vi "DashboardGetvi.vi"(8 "Joystick 2":T1, 9 "Joystick 1":T1) -> ()   [LabVIEW 2018]
uses:
  <vilib>/Rock Robotics/WPI/Joystick/WPI_JoystickDevRef.ctl
  <vilib>/Rock Robotics/WPI/Joystick/WPI_JoystickDeviceEnum.ctl
  <vilib>/Rock Robotics/Network Tables/NT Read Boolean.vi
  <vilib>/Rock Robotics/Network Tables/NT Read Number.vi
  Inputs_DriverStation.vi
  RobotStates.vi
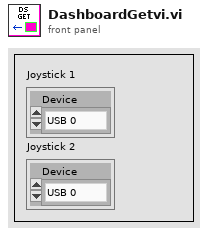
[diagram p1: front panel]
types:
  T1 = typedef "WPI_JoystickDevRef.ctl" = cluster{"Device":T2}
  T2 = typedef "WPI_JoystickDeviceEnum.ctl" = enum16{"USB 0", "USB 1", "USB 2", "USB 3", "USB 4", "USB 5"}
  T3 = cluster{bool, bool, bool, bool, bool, bool, bool, bool, bool, bool, bool, bool, bool, bool}
  T4 = cluster{"Boolean":bool, "Boolean":bool, "Boolean":bool, "Boolean":bool, "Boolean":bool, "Boolean":bool, "Boolean":bool, "Boolean":bool, "Boolean":bool, "Boolean":bool, "Boolean":bool, "Boolean":bool, "Boolean":bool, "Boolean":bool}
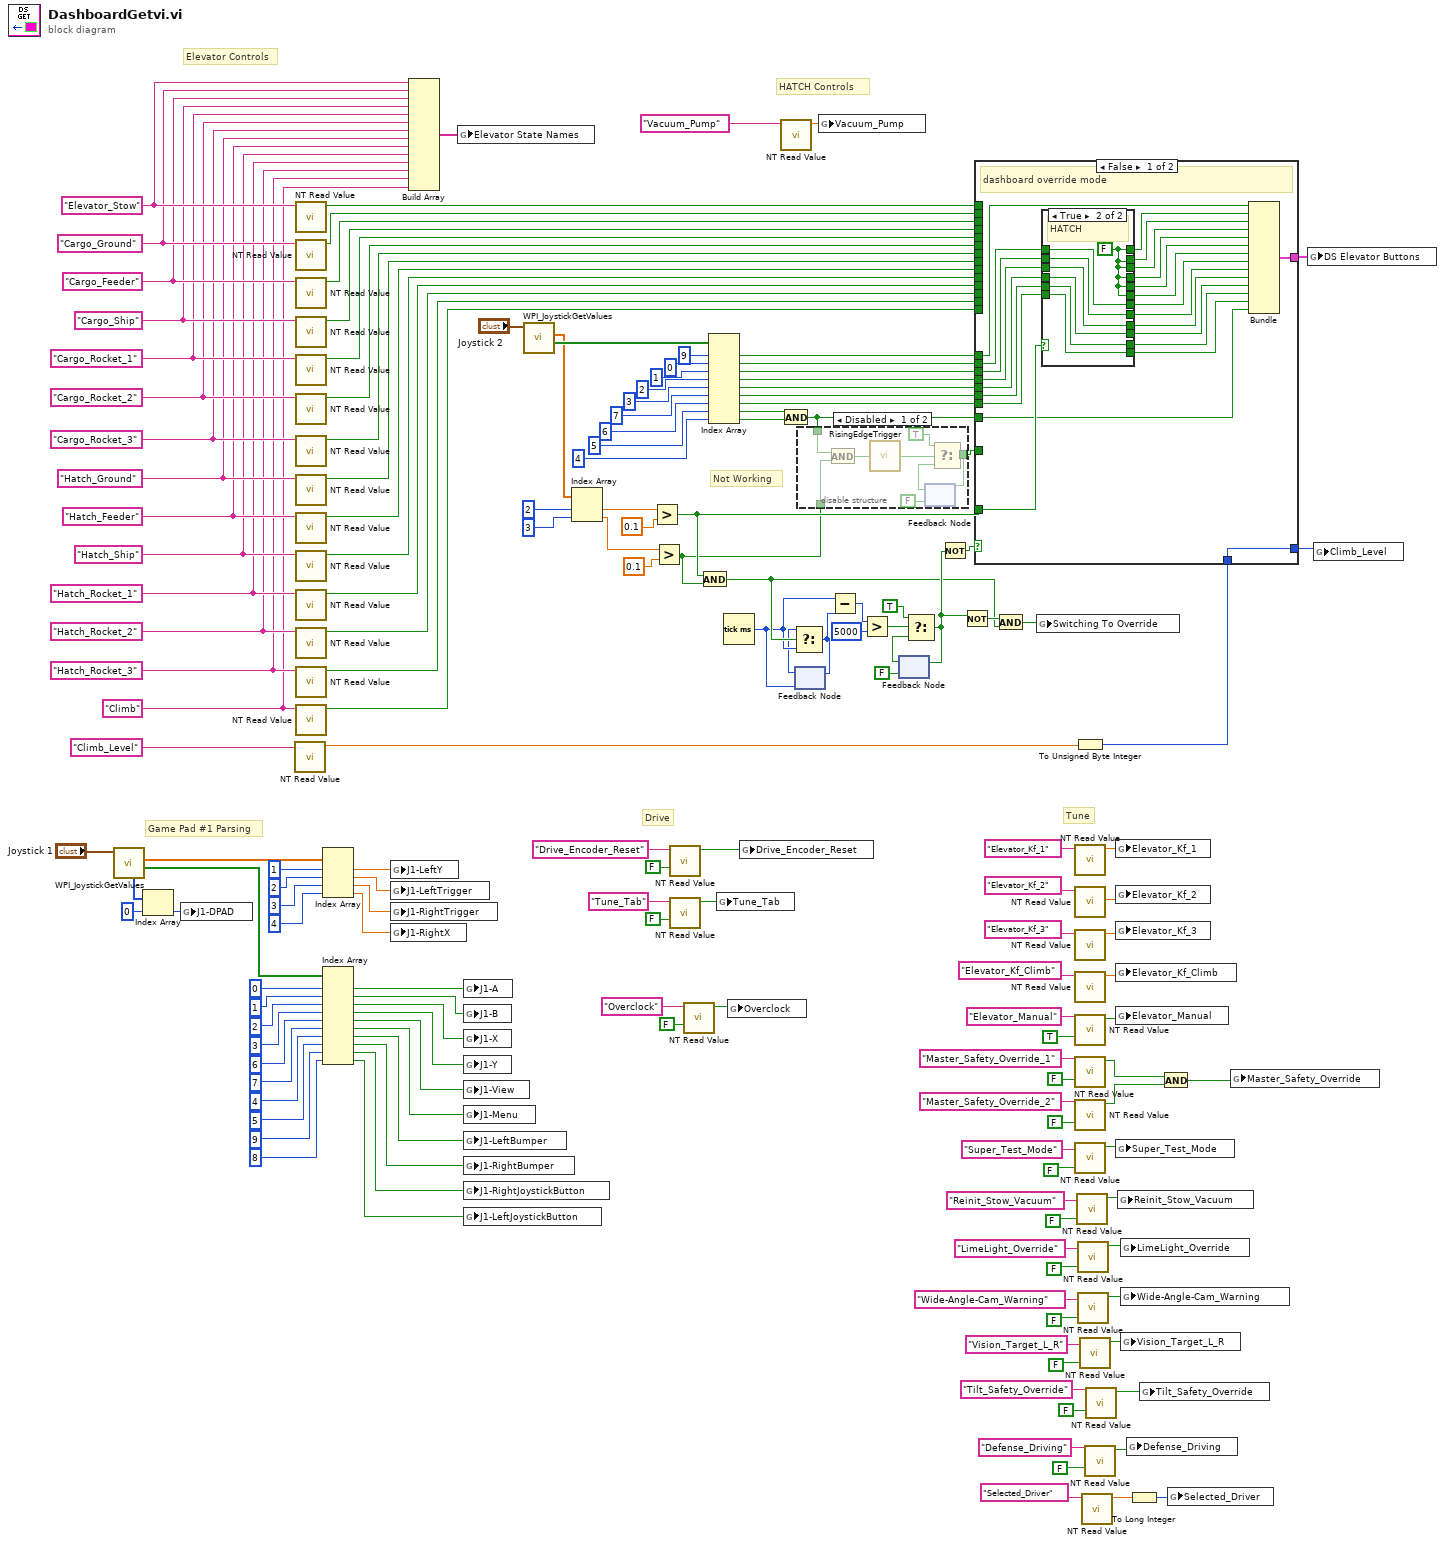
[diagram p0: block diagram]
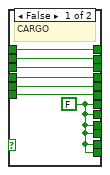
[diagram p3: hidden frame]
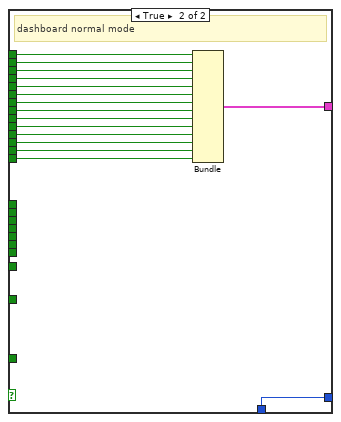
[diagram p4: hidden frame]
diagram:
  w95 = "Climb" ("refnum name")
  w103 = "Hatch_Rocket_3" ("refnum name")
  w104 = "Hatch_Rocket_2" ("refnum name")
  w105 = "Hatch_Rocket_1" ("refnum name")
  w106 = "Hatch_Ship" ("refnum name")
  w107 = "Hatch_Feeder" ("refnum name")
  w108 = "Hatch_Ground" ("refnum name")
  w152 = "Cargo_Rocket_3" ("refnum name")
  w153 = "Cargo_Rocket_2" ("refnum name")
  w154 = "Cargo_Rocket_1" ("refnum name")
  w155 = "Cargo_Ship" ("refnum name")
  w161 = "Cargo_Feeder" ("refnum name")
  w162 = "Cargo_Ground" ("refnum name")
  w163 = "Elevator_Stow" ("refnum name")
  # "Not Working"
  # "Tune"
  # "Drive"
  # "HATCH Controls"
  # "Game Pad #1 Parsing"
  # "Elevator Controls"
  n1 = call <vilib>:"WPI_JoystickGetValues.vi"("JoystickDevRef"="Joystick 1") -> ("Buttons"=w143:bool[], "Axes"=w142:dbl[], "POVs"=w139:i16[])  [unwired: 6 in, 2 out]
  n2 = Index Array(array=w139, index=0) -> (element=w136:i16)
  n3 = global write "Inputs_DriverStation.vi" "J1-DPAD"(w136) -> ()
  n4 = call-poly <vilib>:"NT Read Value.vi"("Name"="Climb_Level" ("refnum name")) -> ("Numeric"=w12:dbl)  [unwired: 9 in, 1 out]
  n5 = call-poly <vilib>:"NT Read Value.vi"("Name"=w163) -> ("Boolean"=w166:bool)  [unwired: 9 in, 1 out]
  n6 = call-poly <vilib>:"NT Read Value.vi"("Name"=w162) -> ("Boolean"=w165:bool)  [unwired: 9 in, 1 out]
  n7 = call-poly <vilib>:"NT Read Value.vi"("Name"=w161) -> ("Boolean"=w164:bool)  [unwired: 9 in, 1 out]
  n8 = call-poly <vilib>:"NT Read Value.vi"("Name"=w155) -> ("Boolean"=w159:bool)  [unwired: 9 in, 1 out]
  n9 = call-poly <vilib>:"NT Read Value.vi"("Name"=w154) -> ("Boolean"=w158:bool)  [unwired: 9 in, 1 out]
  n10 = call-poly <vilib>:"NT Read Value.vi"("Name"=w153) -> ("Boolean"=w157:bool)  [unwired: 9 in, 1 out]
  n11 = call-poly <vilib>:"NT Read Value.vi"("Name"=w152) -> ("Boolean"=w156:bool)  [unwired: 9 in, 1 out]
  n12 = call-poly <vilib>:"NT Read Value.vi"("Name"=w108) -> ("Boolean"=w115:bool)  [unwired: 9 in, 1 out]
  n13 = call-poly <vilib>:"NT Read Value.vi"("Name"=w107) -> ("Boolean"=w114:bool)  [unwired: 9 in, 1 out]
  n14 = call-poly <vilib>:"NT Read Value.vi"("Name"=w106) -> ("Boolean"=w113:bool)  [unwired: 9 in, 1 out]
  n15 = call-poly <vilib>:"NT Read Value.vi"("Name"=w105) -> ("Boolean"=w112:bool)  [unwired: 9 in, 1 out]
  n16 = call-poly <vilib>:"NT Read Value.vi"("Name"=w104) -> ("Boolean"=w111:bool)  [unwired: 9 in, 1 out]
  n17 = call-poly <vilib>:"NT Read Value.vi"("Name"=w103) -> ("Boolean"=w110:bool)  [unwired: 9 in, 1 out]
  n18 = call-poly <vilib>:"NT Read Value.vi"("Name"=w95) -> ("Boolean"=w94:bool)  [unwired: 9 in, 1 out]
  n19 = Index Array(array=w142, index #1=1 ("index"), index #2=2 ("index"), index #3=3 ("index"), index #4=4 ("index")) -> (element #1=w129:dbl, element #2=w130:dbl, element #3=w131:dbl, element #4=w128:dbl)
  n20 = Index Array(array=w143, index #1=0 ("index"), index #2=1 ("index"), index #3=2 ("index"), index #4=3 ("index"), index #5=6 ("index"), index #6=7 ("index"), index #7=4 ("index"), index #8=5 ("index"), index #9=9 ("index"), index #10=8 ("index")) -> (element #1=w135:bool, element #2=w134:bool, element #3=w133:bool, element #4=w132:bool, element #5=w92:bool, element #6=w88:bool, element #7=w85:bool, element #8=w84:bool, element #9=w82:bool, element #10=w77:bool)
  n21 = global write "Inputs_DriverStation.vi" "J1-LeftY"(w129) -> ()
  n22 = global write "Inputs_DriverStation.vi" "J1-LeftTrigger"(w130) -> ()
  n23 = global write "Inputs_DriverStation.vi" "J1-RightTrigger"(w131) -> ()
  n24 = global write "Inputs_DriverStation.vi" "J1-RightX"(w128) -> ()
  n25 = Build Array(w163, w162, w161, w155, w154, w153, w152, w108, w107, w106, w105, w104, w103, w95) -> (w160:string[])
  n26 = global write "RobotStates.vi" "Elevator State Names"(w160) -> ()
  n27 = global write "Inputs_DriverStation.vi" "J1-A"(w135) -> ()
  n28 = global write "Inputs_DriverStation.vi" "J1-B"(w134) -> ()
  n29 = global write "Inputs_DriverStation.vi" "J1-X"(w133) -> ()
  n30 = global write "Inputs_DriverStation.vi" "J1-Y"(w132) -> ()
  n31 = global write "Inputs_DriverStation.vi" "J1-View"(w92) -> ()
  n32 = global write "Inputs_DriverStation.vi" "J1-Menu"(w88) -> ()
  n33 = global write "Inputs_DriverStation.vi" "J1-LeftBumper"(w85) -> ()
  n34 = global write "Inputs_DriverStation.vi" "J1-RightBumper"(w84) -> ()
  n35 = global write "Inputs_DriverStation.vi" "J1-RightJoystickButton"(w82) -> ()
  n36 = global write "Inputs_DriverStation.vi" "J1-LeftJoystickButton"(w77) -> ()
  n37 = call <vilib>:"WPI_JoystickGetValues.vi"("JoystickDevRef"="Joystick 2") -> ("Buttons"=w72:bool[], "Axes"=w56:dbl[])  [unwired: 6 in, 3 out]
  n38 = Index Array(array=w56, index #1=2 ("index"), index #2=3 ("index")) -> (element #1=w55:dbl, element #2=w51:dbl)
  n39 = Greater?(x=w55, y=0.1) -> (0:w50:bool)
  n40 = Greater?(x=w51, y=0.1) -> (0:w38:bool)
  n41 = call-poly <vilib>:"NT Read Value.vi"("Default Value"=FALSE, "Name"="Drive_Encoder_Reset" ("refnum name")) -> ("Boolean"=w116:bool)  [unwired: 8 in, 1 out]
  n42 = call-poly <vilib>:"NT Read Value.vi"("Default Value"=FALSE, "Name"="Tune_Tab" ("refnum name")) -> ("Boolean"=w79:bool)  [unwired: 8 in, 1 out]
  n43 = call-poly <vilib>:"NT Read Value.vi"("Default Value"=FALSE, "Name"="Overclock" ("refnum name")) -> ("Boolean"=w26:bool)  [unwired: 8 in, 1 out]
  n44 = And(x=w50, y=w38) -> (x .and. y?=w32:bool)
  n45 = Index Array(array=w72, index #1=9 ("index"), index #2=0 ("index"), index #3=1 ("index"), index #4=2 ("index"), index #5=3 ("index"), index #6=7 ("index"), index #7=6 ("index"), index #8=5 ("index"), index #9=4 ("index")) -> (element #1=w70:bool, element #2=w68:bool, element #3=w66:bool, element #4=w64:bool, element #5=w62:bool, element #6=w60:bool, element #7=w58:bool, element #8=w41:bool, element #9=w40:bool)
  n46 = global write "Inputs_DriverStation.vi" "Tune_Tab"(w79) -> ()
  n47 = Tick Count (ms)() -> (millisecond timer value=w30:u32)
  n48 = global write "Inputs_DriverStation.vi" "Overclock"(w26) -> ()
  n49 = global write "Inputs_DriverStation.vi" "Drive_Encoder_Reset"(w116) -> ()
  n50 = call-poly <vilib>:"NT Read Value.vi"("Name"="Vacuum_Pump" ("refnum name")) -> ("Numeric"=w119:dbl)  [unwired: 9 in, 1 out]
  n51 = And(x=w41, y=w40) -> (x .and. y?=w39:bool)
  n52 = feedback #1(w30) -> (w29:u32)
  n53 = Select(t=w29, s=w32, f=w30) -> (s? t:f=w36:u32)
  n54 = feedback-in #1(w36) -> ()
  n55 = disable-structure shown="Disabled" {
    disable-tunnel: w39 -> [w174 _]
    disable-tunnel: w38 -> [w173 _]
    disable-tunnel: [w167 _] -> w37
    frame Disabled {
      n56 = And(x=w174, y=w173) -> (x .and. y?=w172:bool)
      n57 = call "RisingEdgeTrigger.vi"("Raw Signal"=w172) -> ("Trigger"=w168:bool)
      n58 = feedback #2(FALSE) -> (w170:bool)
      n59 = Select(t=TRUE, s=w168, f=w170) -> (s? t:f=w167:bool)
      n60 = feedback-in #2(w167) -> ()
    }
    frame Enabled {
    }
  }
  n61 = global write "Inputs_DriverStation.vi" "Vacuum_Pump"(w119) -> ()
  n62 = Subtract(x=w30, y=w36) -> (x-y=w35:u32)
  n63 = Greater?(x=w35, y=u32 5000) -> (0:w48:bool)
  n64 = feedback #3(FALSE) -> (w46:bool)
  n65 = Select(t=TRUE, s=w48, f=w46) -> (s? t:f=w33:bool)
  n66 = feedback-in #3(w33) -> ()
  n67 = Not(x=w33) -> (.not. x?=w44:bool)
  n68 = Not(x=w33) -> (.not. x?=w34:bool)
  n69 = And(x=w34, y=w32) -> (x .and. y?=w31:bool)
  n70 = global write "Inputs_DriverStation.vi" "Switching To Override"(w31) -> ()
  n71 = To Unsigned Byte Integer(number=w12) -> (unsigned 8bit integer=w11:u8)
  n72 = case shown="False" w44 {
    tunnel: w166 -> [_ w227]
    tunnel: w165 -> [_ w226]
    tunnel: w164 -> [_ w225]
    tunnel: w159 -> [_ w224]
    tunnel: w158 -> [_ w223]
    tunnel: w157 -> [_ w222]
    tunnel: w156 -> [_ w221]
    tunnel: w115 -> [_ w220]
    tunnel: w114 -> [_ w219]
    tunnel: w113 -> [_ w218]
    tunnel: w112 -> [_ w217]
    tunnel: w111 -> [_ w216]
    tunnel: w110 -> [_ w215]
    tunnel: [w176 w214] -> w109
    tunnel: w94 -> [_ w213]
    tunnel: w70 -> [w197 _]
    tunnel: w68 -> [w196 _]
    tunnel: w66 -> [w194 _]
    tunnel: w64 -> [w192 _]
    tunnel: w62 -> [w191 _]
    tunnel: w60 -> [w190 _]
    tunnel: w58 -> [w189 _]
    tunnel: w50 -> [w188 _]
    tunnel: w39 -> [w187 _]
    tunnel: [w175 w212] -> w10
    tunnel: w37 -> [_ _]
    tunnel: w11 -> [w175 w212]
    frame False {
      # "dashboard override mode"
      n73 = case shown="True" w188 {
        tunnel: w196 -> [w204 w210]
        tunnel: [w204 w211] -> w195
        tunnel: w194 -> [w203 w209]
        tunnel: [w203 w211] -> w193
        tunnel: w192 -> [w202 w208]
        tunnel: [w202 w211] -> w186
        tunnel: w191 -> [w201 w207]
        tunnel: [w201 w211] -> w185
        tunnel: w190 -> [w200 w206]
        tunnel: [w200 w211] -> w184
        tunnel: w189 -> [w199 w205]
        tunnel: [w199 w211] -> w183
        tunnel: [w198 w210] -> w182
        tunnel: [w198 w209] -> w181
        tunnel: [w198 w208] -> w180
        tunnel: [w198 w207] -> w179
        tunnel: [w198 w206] -> w178
        tunnel: [w198 w205] -> w177
        frame False {
          w198 = FALSE
          # "CARGO"
        }
        frame True {
          w211 = FALSE
          # "HATCH"
        }
      }
      n74 = Bundle(w197, w195, w193, w186, w185, w184, w183, w182, w181, w180, w179, w178, w177, w187) -> (w176:T3)  [unwired: 1 in]
    }
    frame True {
      # "dashboard normal mode"
      n75 = Bundle("Boolean"=w227, "Boolean"=w226, "Boolean"=w225, "Boolean"=w224, "Boolean"=w223, "Boolean"=w222, "Boolean"=w221, "Boolean"=w220, "Boolean"=w219, "Boolean"=w218, "Boolean"=w217, "Boolean"=w216, "Boolean"=w215, "Boolean"=w213) -> (w214:T4)  [unwired: 1 in]
    }
  }
  n76 = call-poly <vilib>:"NT Read Value.vi"("Name"="Elevator_Kf_1" ("refnum name")) -> ("Numeric"=w150:dbl)  [unwired: 9 in, 1 out]
  n77 = call-poly <vilib>:"NT Read Value.vi"("Name"="Elevator_Kf_2" ("refnum name")) -> ("Numeric"=w123:dbl)  [unwired: 9 in, 1 out]
  n78 = call-poly <vilib>:"NT Read Value.vi"("Name"="Elevator_Kf_3" ("refnum name")) -> ("Numeric"=w121:dbl)  [unwired: 9 in, 1 out]
  n79 = call-poly <vilib>:"NT Read Value.vi"("Name"="Elevator_Kf_Climb" ("refnum name")) -> ("Numeric"=w90:dbl)  [unwired: 9 in, 1 out]
  n80 = call-poly <vilib>:"NT Read Value.vi"("Default Value"=TRUE, "Name"="Elevator_Manual" ("refnum name")) -> ("Boolean"=w126:bool)  [unwired: 8 in, 1 out]
  n81 = call-poly <vilib>:"NT Read Value.vi"("Default Value"=FALSE, "Name"="Master_Safety_Override_1" ("refnum name")) -> ("Boolean"=w98:bool)  [unwired: 8 in, 1 out]
  n82 = call-poly <vilib>:"NT Read Value.vi"("Default Value"=FALSE, "Name"="Master_Safety_Override_2" ("refnum name")) -> ("Boolean"=w97:bool)  [unwired: 8 in, 1 out]
  n83 = call-poly <vilib>:"NT Read Value.vi"("Default Value"=FALSE, "Name"="Super_Test_Mode" ("refnum name")) -> ("Boolean"=w75:bool)  [unwired: 8 in, 1 out]
  n84 = call-poly <vilib>:"NT Read Value.vi"("Default Value"=FALSE, "Name"="Reinit_Stow_Vacuum" ("refnum name")) -> ("Boolean"=w24:bool)  [unwired: 8 in, 1 out]
  n85 = call-poly <vilib>:"NT Read Value.vi"("Default Value"=FALSE, "Name"="LimeLight_Override" ("refnum name")) -> ("Boolean"=w21:bool)  [unwired: 8 in, 1 out]
  n86 = call-poly <vilib>:"NT Read Value.vi"("Default Value"=FALSE, "Name"="Wide-Angle-Cam_Warning" ("refnum name")) -> ("Boolean"=w17:bool)  [unwired: 8 in, 1 out]
  n87 = call-poly <vilib>:"NT Read Value.vi"("Default Value"=FALSE, "Name"="Vision_Target_L_R" ("refnum name")) -> ("Boolean"=w14:bool)  [unwired: 8 in, 1 out]
  n88 = call-poly <vilib>:"NT Read Value.vi"("Name"="Selected_Driver" ("refnum name")) -> ("Numeric"=w2:dbl)  [unwired: 9 in, 1 out]
  n89 = call-poly <vilib>:"NT Read Value.vi"("Default Value"=FALSE, "Name"="Defense_Driving" ("refnum name")) -> ("Boolean"=w5:bool)  [unwired: 8 in, 1 out]
  n90 = call-poly <vilib>:"NT Read Value.vi"("Default Value"=FALSE, "Name"="Tilt_Safety_Override" ("refnum name")) -> ("Boolean"=w7:bool)  [unwired: 8 in, 1 out]
  n91 = global write "Inputs_DriverStation.vi" "Elevator_Kf_1"(w150) -> ()
  n92 = global write "Inputs_DriverStation.vi" "Elevator_Kf_2"(w123) -> ()
  n93 = global write "Inputs_DriverStation.vi" "Elevator_Kf_3"(w121) -> ()
  n94 = global write "Inputs_DriverStation.vi" "Elevator_Kf_Climb"(w90) -> ()
  n95 = global write "Inputs_DriverStation.vi" "Elevator_Manual"(w126) -> ()
  n96 = global write "Inputs_DriverStation.vi" "Super_Test_Mode"(w75) -> ()
  n97 = global write "Inputs_DriverStation.vi" "Reinit_Stow_Vacuum"(w24) -> ()
  n98 = global write "Inputs_DriverStation.vi" "LimeLight_Override"(w21) -> ()
  n99 = global write "Inputs_DriverStation.vi" "Wide-Angle-Cam_Warning"(w17) -> ()
  n100 = global write "Inputs_DriverStation.vi" "Vision_Target_L_R"(w14) -> ()
  n101 = global write "Inputs_DriverStation.vi" "Defense_Driving"(w5) -> ()
  n102 = To Long Integer(number=w2) -> (32bit integer=w1:i32)
  n103 = global write "Inputs_DriverStation.vi" "Tilt_Safety_Override"(w7) -> ()
  n104 = And(x=w98, y=w97) -> (x .and. y?=w96:bool)
  n105 = global write "Inputs_DriverStation.vi" "Selected_Driver"(w1) -> ()
  n106 = global write "Inputs_DriverStation.vi" "Master_Safety_Override"(w96) -> ()
  n107 = global write "Inputs_DriverStation.vi" "DS Elevator Buttons"(w109) -> ()
  n108 = global write "Inputs_DriverStation.vi" "Climb_Level"(w10) -> ()
